vi "test_hts_commands.vi"() -> ()   [LabVIEW 2013]
uses:
  main_machine/type_defs/global_settings.ctl
  main_machine/type_defs/experiment_settings.ctl
  main_machine/type_defs/experiment_states.ctl
  hts/type_defs/hts_command_list.ctl
  <vilib>/Utility/file.llb/Read From Spreadsheet File (DBL).vi
panel:
  out "all rows":dbl[][](array[numeric]) format="%0.3f"
  in  "Error IN":errorcluster
  in  "COMMAND":T1=enum."REMOVE CULTURE"
  in  "EXPERIMENT SETTINGS":T2={"fcs file byte offset"=0, "LED Device Handle Out"=0, "START TIME"=timestamp(0 s since 1904-01-01), "CURRENT VALVE"=0, "SAMPLE #"=0, "FCS FILE PATH"=path "", "TIME POINT"=1, "STATE"=enum."EXPERIMENT", "TIME TILL SAMPLE"=0.0, "DILUTION  TABLE"=[]}
  in  "SETTINGS":T4={"# REACTORS"=8, "17X PORT"=9, "WASTE POSITION "=3, "SECONDS BETWEEN SAMPLING"=1440.0, "FACS DIVA DIRECTORY"=path "D:/BDDatabase/BDData", "DATA FILE"=path "C:/Documents and Settings/HES/Desktop/THN20180328_datafiletest.csv", "REACTORS TO USE"=[5, 4, 7, 6, 11, 1, 2, 12], "PULSE PERIOD"=120, "USE LIGHTS?"=TRUE, "LED FILE"=path "C:/Documents and Settings/HES/Desktop/THN20180327_lightfile.csv", "LED CHANNELS"=[3, 4, 2, 1, 8, 7, 6, 5], "PULSE LENGTH"=1, "SUMMARY FILE"=path "C:/Documents and Settings/HES/Desktop/THN20180328_summaryfiletest.csv", "OUTGROWTH TIME POINTS"=0.0, "SELECTION VALVE PORT"="COM4", "HTS PORT"="COM5", "DILUTION VOLUME (uL)"=3500, "DILUTION FILE"=path "C:/Documents and Settings/HES/Desktop/THN20180327_dilutionfile.csv", "1X PORT"=8}
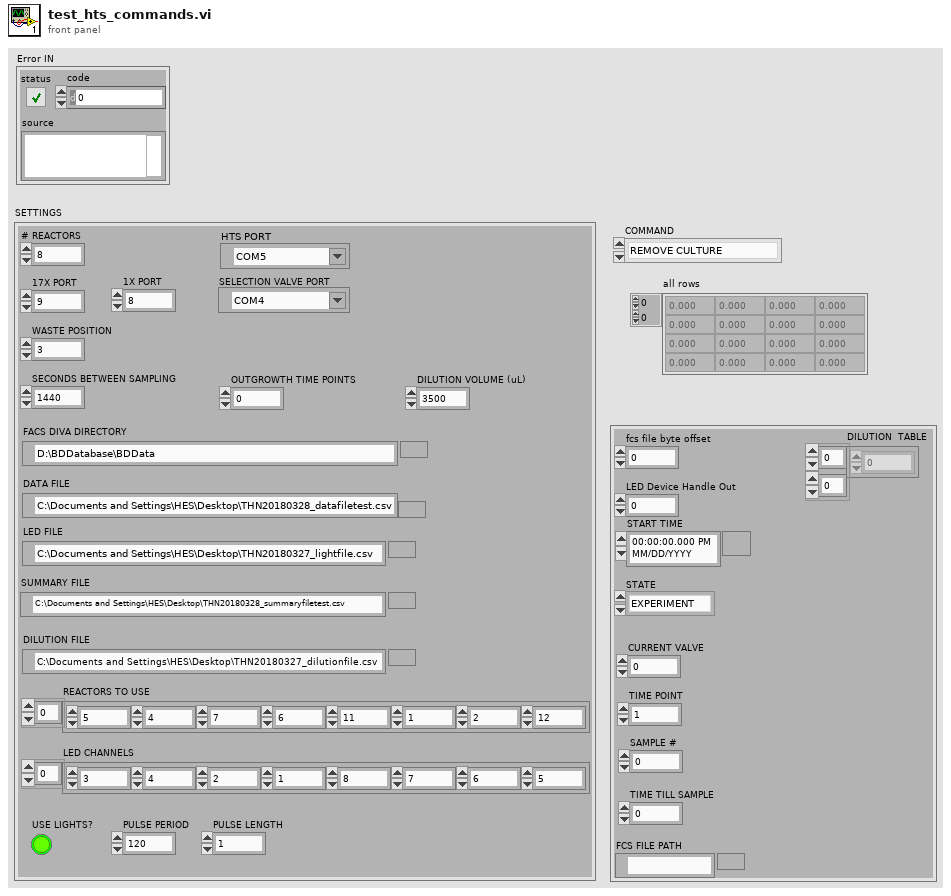
[diagram p1: front panel]
types:
  T1 = typedef "hts_command_list.ctl" = enum16{"INITIALIZE", "ADD MEDIA", "ADD INDUCER", "REMOVE CULTURE", "SAMPLE REACTOR", "CLEAR LINE TO VALVE", "CLEAR LINE TO CYTOMETER"}
  T2 = typedef "experiment_settings.ctl" = cluster{"fcs file byte offset":i64, "LED Device Handle Out":u32, "START TIME":timestamp, "CURRENT VALVE":u32, "SAMPLE #":i32, "FCS FILE PATH":path, "TIME POINT":i32, "STATE":T3, "TIME TILL SAMPLE":dbl, "DILUTION  TABLE":dbl[][]}
  T3 = typedef "experiment_states.ctl" = enum16{"OUTGROWTH", "INDUCTION", "EXPERIMENT"}
  T4 = typedef "global_settings.ctl" = cluster{"# REACTORS":u32, "17X PORT":i32, "WASTE POSITION ":i32, "SECONDS BETWEEN SAMPLING":dbl, "FACS DIVA DIRECTORY":path, "DATA FILE":path, "REACTORS TO USE":u32[], "PULSE PERIOD":i32, "USE LIGHTS?":bool, "LED FILE":path, "LED CHANNELS":u32[], "PULSE LENGTH":i32, "SUMMARY FILE":path, "OUTGROWTH TIME POINTS":dbl, "SELECTION VALVE PORT":refnum<visa-resource-name>, "HTS PORT":refnum<visa-resource-name>, "DILUTION VOLUME (uL)":i32, "DILUTION FILE":path, "1X PORT":i32}
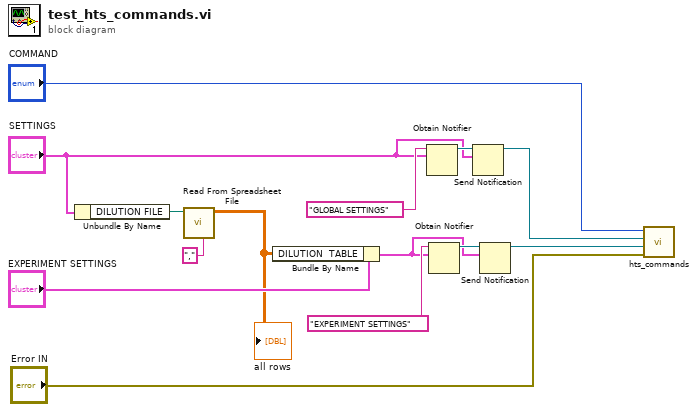
[diagram p0: block diagram]
diagram:
  n1 = Unbundle By Name("SETTINGS") -> ("DILUTION FILE"=w14:path)
  n2 = call-poly <vilib>:"Read From Spreadsheet File.vi"("delimiter (\\t)"="," ("delimiter (\\t)"), "file path (dialog if empty)"=w14) -> ("all rows"=w11:dbl[][])  [unwired: 5 in, 4 out]
  "all rows" <- w11
  n3 = Bundle By Name(cluster="EXPERIMENT SETTINGS", "DILUTION  TABLE"=w11) -> (w1:T2)
  n4 = Obtain Notifier(name (unnamed)="GLOBAL SETTINGS", notification data type="SETTINGS") -> (notifier out=w6:refnum<notifier>)  [unwired: 2 in, 2 out]
  n5 = Obtain Notifier(name (unnamed)="EXPERIMENT SETTINGS", notification data type=w1) -> (notifier out=w3:refnum<notifier>)  [unwired: 2 in, 2 out]
  n6 = Send Notification(notification="SETTINGS", notifier=w6) -> (notifier out=w5:refnum<notifier>)  [unwired: 1 in, 1 out]
  n7 = Send Notification(notification=w1, notifier=w3) -> (notifier out=w2:refnum<notifier>)  [unwired: 1 in, 1 out]
  n8 = call "hts_commands.vi"("Error IN"="Error IN", "EXP SETTINGS"=w2, "SETTINGS"=w5, "COMMAND"="COMMAND") -> ()  [unwired: 5 in, 3 out]
